vi "Read Acquisition start.vi"(8 "error in (no error)":errorcluster, 11 "Acquis params in":refnum<class "CV-Acquisition.lvclass">) -> (0 "error out":errorcluster, 2 "Acquisition start":enum16{"Immediate", "Post-phoned"}(ring), 3 "Acquis params out":refnum<class "CV-Acquisition.lvclass">)   [LabVIEW 2013, in "CameraVision.lvlib" / "CV-Acquisition.lvclass"]
uses:
  CV-Acquisition.lvclass
  CV-Acquisition.lvclass/CV-Acquisition.ctl
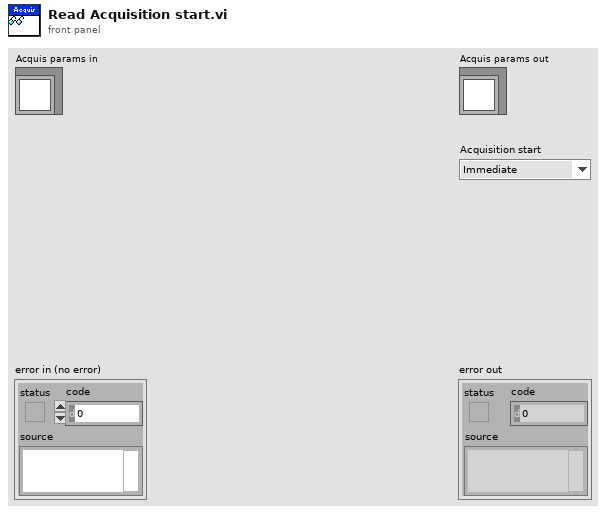
[diagram p1: front panel]
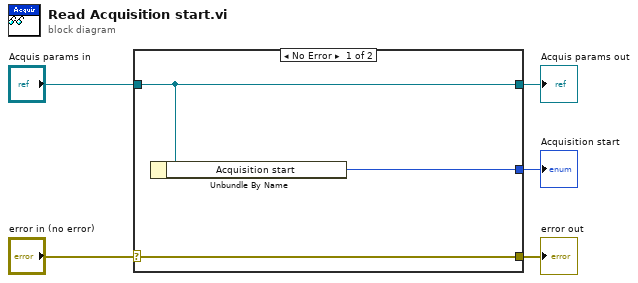
[diagram p0: block diagram]
diagram:
  n1 = case shown="No Error" "error in (no error)" {
    selector: "error in (no error)" -> [w8 w9]
    tunnel: [w8 w9] -> w4
    tunnel: [w7 w10] -> w2
    tunnel: "Acquis params in" -> [w7 w10]
    tunnel: [w6 _] -> w1
    frame No Error {
      n2 = Unbundle By Name(w7) -> ("Acquisition start"=w6:enum16{"Immediate", "Post-phoned"})
    }
    frame Error {
    }
  }
  "error out" <- w4
  "Acquis params out" <- w2
  "Acquisition start" <- w1
